vi "Get Report Path.vi"(8 "error in (no error)":errorcluster, 11 "Configuration Manager in":refnum<class "Configuration Manager.lvclass">) -> (0 "error out":errorcluster, 2 "Report Path":path, 3 "Configuration Manager out":refnum<class "Configuration Manager.lvclass">)   [LabVIEW 2020, in "Configuration Manager.lvclass"]
uses:
  Configuration Manager.lvclass
  Configuration Manager.lvclass/Configuration Manager.ctl
  <vilib>/Utility/config.llb/Read Key (Path).vi
  <vilib>/Utility/config.llb/NI_LVConfig.lvlib
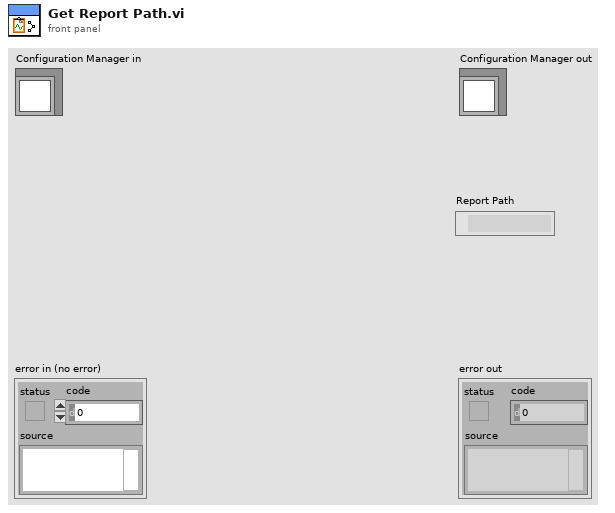
[diagram p1: front panel]
types:
  T1 = typedef "NI_LVConfig.lvlib/Config Data RefNum.ctl" = refnum<k1>
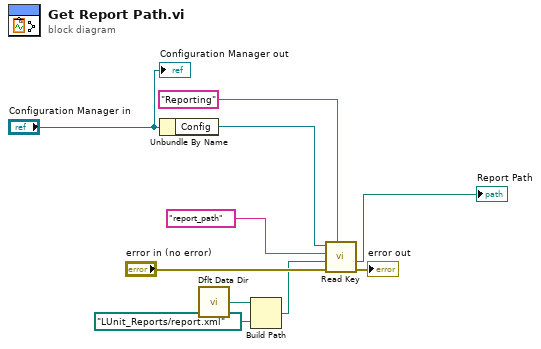
[diagram p0: block diagram]
diagram:
  n1 = Unbundle By Name("Configuration Manager in") -> ("Config"=w9:T1)
  n2 = call <vilib>:"Dflt Data Dir.vi"() -> ("App:Default Data Directory"=w5:path)
  n3 = Build Path(base path=w5, name or relative path=path "LUnit_Reports/report.xml") -> (appended path=w3:path)
  n4 = call-poly <vilib>:"Read Key.vi"("section"="Reporting", "error in (no error)"="error in (no error)", "default value"=w3, "key"="report_path", "refnum"=w9) -> ("error out"=→"error out":errorcluster, "value"=→"Report Path":path)  [unwired: 3 in, 2 out]
  "Configuration Manager out" <- "Configuration Manager in"
